vi "CRYGet Hardware Info From Signal Type.vi"(8 "Calibration In":string, 9 "Hardware In":string, 10 "Signal Type":string, 11 "In/Out?":bool) -> (1 "Channel Array Index":i32, 2 "Exist?":bool, 3 "Channel Info Out":T1={"ID"=0, "Name"="", "Digital"=FALSE, "Input"=FALSE, "Device Name"="", "Hardware Ch ID"=0, "Vmax (V)"=0.0, "Latency (samples)"=0.0, "Sampling Rate (Hz)"=0, "Bit Depth"=0, "Anti-aliasing Factor (%fs)"=0.0, "DAQmx Channel"="", "term config"=-1, "Coupling"=0, "IEPE en"=FALSE, "ASIOChannel Name"="", "Audio Driver"=0, "ASIOChannel Index"=0} {"Coupling" items=["Default"=-1, "RSE"=10083, "NRSE"=10078, "Differential"=10106, "Pseudodifferential"=12529]; "term config" items=["Default"=-1, "RSE"=10083, "NRSE"=10078, "Differential"=10106, "Pseudodifferential"=12529]; "Anti-aliasing Factor (%fs)" format="%.2f"})   [LabVIEW 2013]
uses:
  Typedef Control/CRYHardware Channel Info.ctl
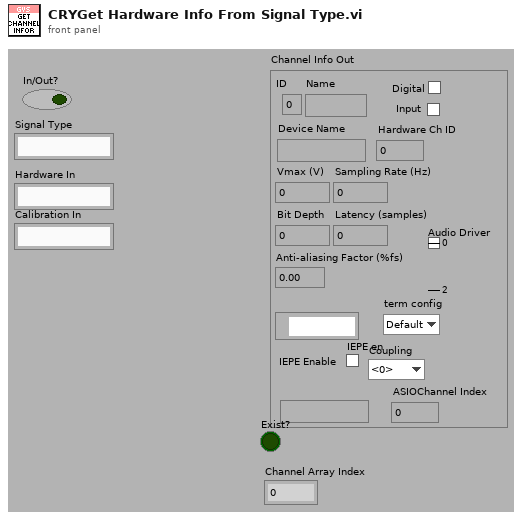
[diagram p1: front panel]
types:
  T1 = typedef "CRYHardware Channel Info.ctl" = cluster{"ID":i32, "Name":string, "Digital":bool, "Input":bool, "Device Name":string, "Hardware Ch ID":u8, "Vmax (V)":dbl, "Latency (samples)":dbl, "Sampling Rate (Hz)":u32, "Bit Depth":u32, "Anti-aliasing Factor (%fs)":sgl, "DAQmx Channel":tag, "term config":i32, "Coupling":i32, "IEPE en":bool, "ASIOChannel Name":string, "Audio Driver":u16, "ASIOChannel Index":u8}
  T2 = typedef "CRYCalibration All Cluster.ctl" = cluster{"Calibration 2D":T3[], "Help":string, "Tab Value":i32, "Input Signal Type":string, "Output Signal Type":string}
  T3 = typedef "CRYCalibration 2DCluster.ctl" = cluster{"Calibration":T4, "Corr Curve":T5, "EQ Curve":T5, "Sens Curve":T5}
  T4 = typedef "CRYCalibration Cluster.ctl" = cluster{"Calibration Step Name":string, "Device":string, "Correction Curve Name":string, "Equalization Curve Name":string, "Sensitivity Curve Name":string, "Corr Folder and File":string, "EQ Folder and File":string, "Sens Folder and File":string, "Corr Step size":u16, "EQ Step size":u16, "Input":bool, "Last Cal Date (sec)":timestamp, "Cha Name":string, "Corr Curve Found":bool, "EQ Curve Found":bool, "Sens Curve Found":bool, "Signal Type":string, "Calibrated Device":string, "Hz":u32}
  T5 = typedef "CRYData Cluster.ctl" = cluster{"Name":string, "Curve":cluster{"x":dbl, "y":dbl, "z":dbl}[], "X data":u16, "Y data":u16, "Z data":u16, "X axis":u16, "Y axis":u16, "Z axis":u16, "X unit":string, "Y unit":string, "Z unit":string, "X dB ref":dbl, "Y dB ref":dbl, "Z dB ref":dbl, "single val":bool, "protected":bool, "display X":bool, "display Y":bool, "display Z":bool, "Test Info":string, "Step No.":i32, "Plot Settings":cluster{"Color":u32, "Interpolation":u8, "Point Style":u8, "Line Style":u8, "Point Color":u32, "Line Width":u8, "Bar Plot Style":u8, "Fill To":i16}, "AutoProtect":bool}
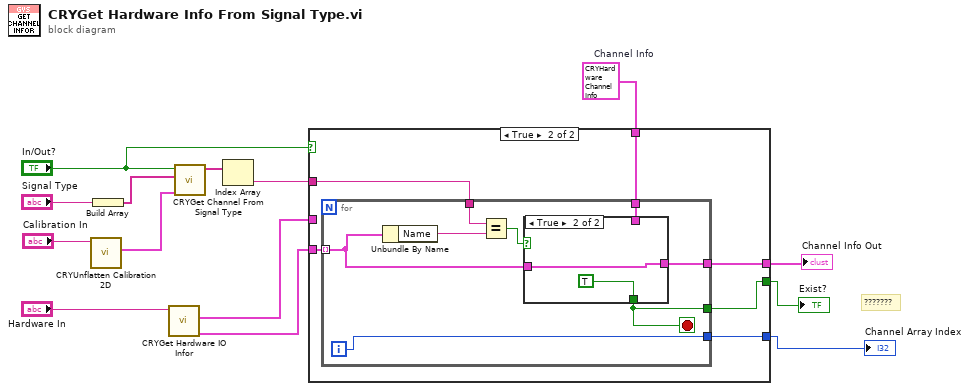
[diagram p0: block diagram]
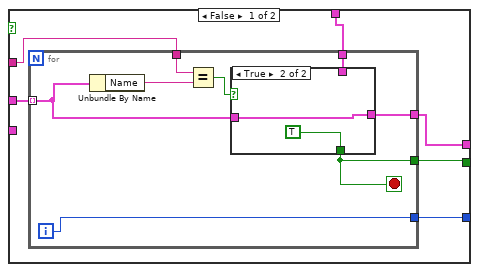
[diagram p2: hidden frame]
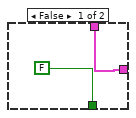
[diagram p3: hidden frame]
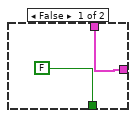
[diagram p4: hidden frame]
diagram:
  w11 = T1 {"ID"=0, "Name"="", "Digital"=FALSE, "Input"=FALSE, "Device Name"="", "Hardware Ch ID"=0, "Vmax (V)"=0.0, "Latency (samples)"=0.0, "Sampling Rate (Hz)"=0, "Bit Depth"=0, "Anti-aliasing Factor (%fs)"=0.475, "DAQmx Channel"="", "term config"=0, "Coupling"=-1, "IEPE en"=FALSE, "ASIOChannel Name"="", "Audio Driver"=0, "ASIOChannel Index"=0}  # Channel Info
  # "???????"
  n1 = call "CRYUnflatten Calibration 2D.vi"("Flattened Calibration"="Calibration In") -> ("Calibration Step Out"=w3:T2)  [unwired: 8 in, 2 out]
  n2 = Build Array("Signal Type") -> (w9:string[])
  n3 = call "CRYGet Hardware IO Infor.vi"("Hardware setup In"="Hardware In") -> ("I_channel Info Out"=w13:T1[], "O_channel Info Out"=w5:T1[])  [unwired: 9 out]
  n4 = call "CRYGet Channel From Signal Type.vi"("Calibration"=w3, "Signal Type Name Array In"=w9, "In/Out?"="In/Out?") -> ("Channel Name Array Out"=w8:string[])  [unwired: 7 in, 1 out]
  n5 = Index Array(array=w8) -> (element=w7:string)  [unwired: 1 in]
  n6 = case shown="True" "In/Out?" {
    tunnel: w13 -> [_ w38]
    tunnel: [w17 w37] -> w12
    tunnel: w11 -> [w18 w36]
    tunnel: w7 -> [w19 w35]
    tunnel: w5 -> [w20 _]
    tunnel: [w16 w34] -> w2
    tunnel: [w15 w33] -> w1
    frame False {
      n7 = for {
        tunnel: w20 -> [w24] mode=indexing
        tunnel: [w28] -> w17
        tunnel: w19 -> [w27]
        tunnel: w18 -> [w23]
        tunnel: [w22] -> w16
        tunnel: [w21] -> w15
        i -> [w21]
        stop <- w22 stop-if-true
        n8 = Unbundle By Name(w24) -> ("Name"=w26:string)
        n9 = Equal?(x=w27, y=w26) -> (x = y?=w25:bool)
        n10 = case shown="True" w25 {
          tunnel: [FALSE TRUE] -> w22
          tunnel: [w29 w31] -> w28
          tunnel: w24 -> [_ w31]
          tunnel: w23 -> [w29 _]
          frame False {
          }
          frame True {
          }
        }
      }
    }
    frame True {
      n11 = for {
        tunnel: w38 -> [w42] mode=indexing
        tunnel: [w46] -> w37
        tunnel: w35 -> [w45]
        tunnel: w36 -> [w41]
        tunnel: [w40] -> w34
        tunnel: [w39] -> w33
        i -> [w39]
        stop <- w40 stop-if-true
        n12 = Unbundle By Name(w42) -> ("Name"=w44:string)
        n13 = Equal?(x=w45, y=w44) -> (x = y?=w43:bool)
        n14 = case shown="True" w43 {
          tunnel: [FALSE TRUE] -> w40
          tunnel: [w47 w49] -> w46
          tunnel: w42 -> [_ w49]
          tunnel: w41 -> [w47 _]
          frame False {
          }
          frame True {
          }
        }
      }
    }
  }
  "Channel Info Out" <- w12
  "Exist?" <- w2
  "Channel Array Index" <- w1
